vi "(a+b)2.vi"() -> ()   [LabVIEW 2015]
panel:
  out "Boolean":bool
  in  "Numeric 2":dbl
  in  "Numeric":dbl
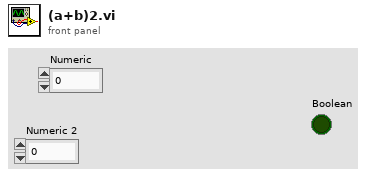
[diagram p1: front panel]
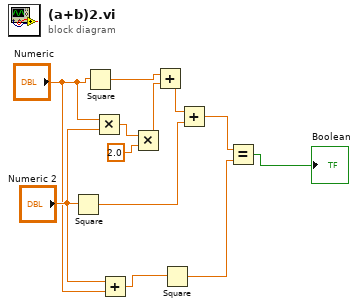
[diagram p0: block diagram]
diagram:
  n1 = Square(x="Numeric 2") -> (x^2=w7:dbl)
  n2 = Square(x="Numeric") -> (x^2=w10:dbl)
  n3 = Multiply(x="Numeric", y="Numeric 2") -> (x*y=w12:dbl)
  n4 = Add(x="Numeric 2", y="Numeric") -> (x+y=w3:dbl)
  n5 = Multiply(x=w12, y=2.0 ("Numeric 3")) -> (x*y=w9:dbl)
  n6 = Add(x=w10, y=w9) -> (x+y=w8:dbl)
  n7 = Square(x=w3) -> (x^2=w2:dbl)
  n8 = Add(x=w8, y=w7) -> (x+y=w6:dbl)
  n9 = Equal?(x=w6, y=w2) -> (x = y?=→"Boolean":bool)
